vi "ex_XColumnsText.vi"(7 "file info in":T1={"delimiter"="\t", "origin time"=timestamp(0 s since 1904-01-01), "Flags"={"include col headings?"=TRUE, "x_columns"=0, "col headings always?"=TRUE, "time preference"=0, "hide col headings"=FALSE}, "Decimal Separator"=""} {"Flags"."time preference" items=["Absolute", "Relative"]; "Flags"."x_columns" items=["None", "One", "Multiple"]; "origin time" format="%<%X\n%x>T"}) -> (1 "xcolumns":string, 3 "file info out":T1={"delimiter"="\t", "origin time"=timestamp(0 s since 1904-01-01), "Flags"={"include col headings?"=TRUE, "x_columns"=0, "col headings always?"=TRUE, "time preference"=0, "hide col headings"=FALSE}, "Decimal Separator"=""} {"Flags"."time preference" items=["Absolute", "Relative"]; "Flags"."x_columns" items=["None", "One", "Multiple"]; "origin time" format="%<%X\n%x>T"})   [LabVIEW 2020]
uses:
  ex_WriteFileParams.ctl
  express input/ExFileReadBlock.llb/ex_ReadFileParams.ctl
panel:
  in  "x_columns":u16(ring) items=["None", "One", "Multiple"]
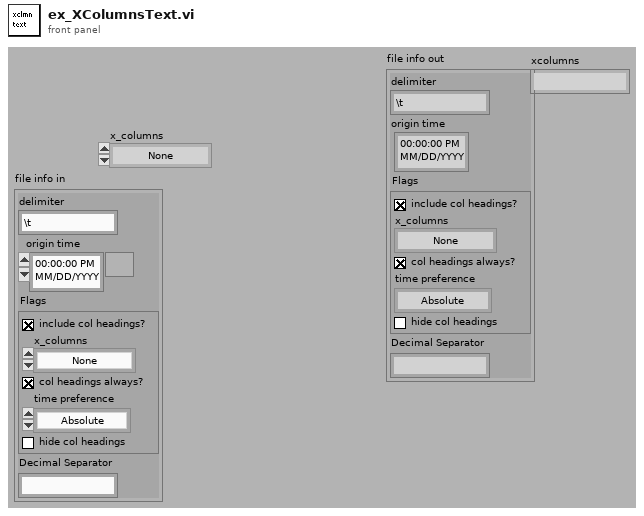
[diagram p1: front panel]
types:
  T1 = typedef "ex_WriteFileParams.ctl" = cluster{"delimiter":string, "origin time":timestamp, "Flags":T2, "Decimal Separator":string}
  T2 = typedef "ex_ReadFileParams.ctl" = cluster{"include col headings?":bool, "x_columns":u16, "col headings always?":bool, "time preference":u16, "hide col headings":bool}
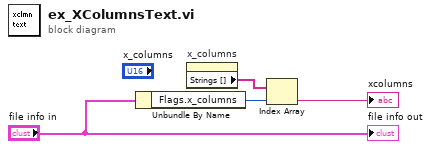
[diagram p0: block diagram]
diagram:
  n1 = Unbundle By Name("file info in") -> ("Flags.x_columns"=w3:u16)
  n2 = property on="x_columns" class="Ring (strict)"() -> ("Strings []"=w4:string[])  [unwired: 2 in, 2 out]
  n3 = Index Array(array=w4, index=w3) -> (element=→"xcolumns":string)
  "file info out" <- "file info in"
